vi "Sphere.vi"(4 "Position":cluster{"X":sgl, "Y":sgl, "Z":sgl}, 5 "Alpha":dbl=1.0, 6 "Detail":sgl=1.0, 7 "Color Box":u32(colorbox), 8 "error in (no error)":errorcluster, 9 "Radius":sgl=1.0, 10 "Name":string) -> (0 "error out":errorcluster, 3 "3D Object out":refnum<class "3D Object.lvclass">)   [LabVIEW 2015, in "3D Object.lvclass"]
uses:
  3D Object.lvclass
  <vilib>/picture/3D Picture Control/NI_3D Picture Control.lvlib
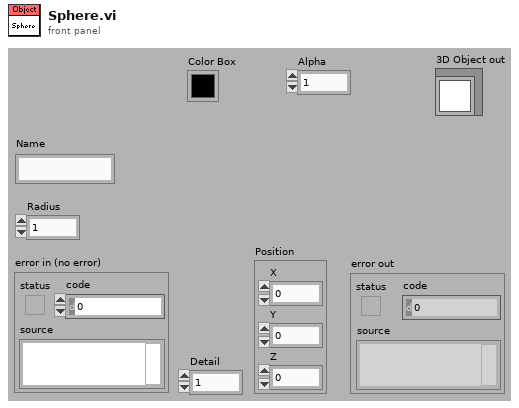
[diagram p1: front panel]
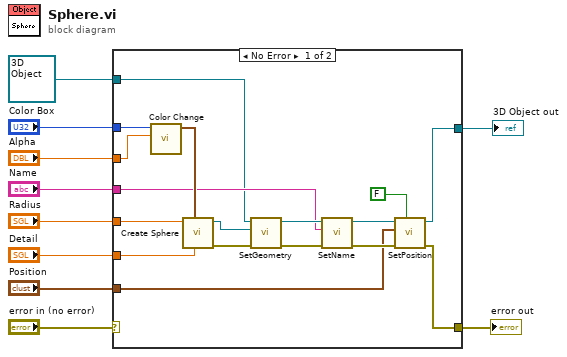
[diagram p0: block diagram]
diagram:
  n1 = case shown="No Error" "error in (no error)" {
    selector: "error in (no error)" -> [_ w28]
    tunnel: "Color Box" -> [w26 _]
    tunnel: "Alpha" -> [w25 _]
    tunnel: "Radius" -> [w24 _]
    tunnel: "Detail" -> [w23 _]
    tunnel: refnum<class "3D Object.lvclass"> refnum ("3D Object in") -> [w13 w29]
    tunnel: [w20 w29] -> w4
    tunnel: [w19 w28] -> w3
    tunnel: "Position" -> [w12 _]
    tunnel: "Name" -> [w14 _]
    frame No Error {
      n2 = call <vilib>:"Color Change.vi"("Alpha"=w25, "Color"=w26) -> ("RGBA"=w27:cluster{"R":sgl, "G":sgl, "B":sgl, "A":sgl})  [unwired: 9 out]
      n3 = call <vilib>:"Create Sphere.vi"("Detail"=w23, "Color"=w27, "Radius"=w24) -> ("error out"=w22:errorcluster, "New Sphere Refnum"=w21:refnum<vi>)  [unwired: 1 in, 6 out]
      n4 = call "SetGeometry.vi"("error in (no error)"=w22, "Geometry"=w21, "Object in"=w13) -> ("error out"=w17:errorcluster, "Object out"=w18:refnum<class "3D Object.lvclass">)  [unwired: 7 out]
      n5 = call "SetName.vi"("error in (no error)"=w17, "Name"=w14, "3D Object in"=w18) -> ("error out"=w15:errorcluster, "3D Object out"=w16:refnum<class "3D Object.lvclass">)  [unwired: 7 out]
      n6 = call "SetPosition.vi"("Relative?"=FALSE, "error in (no error)"=w15, "Position"=w12, "3D Object in"=w16) -> ("error out"=w19:errorcluster, "3D Object out"=w20:refnum<class "3D Object.lvclass">)  [unwired: 6 in]
    }
    frame Error {
    }
  }
  "error out" <- w3
  "3D Object out" <- w4
